vi "new-id.vi"(8 "error in (no error)":errorcluster, 10 "id-string (\"\": generate new id)":string) -> (0 "error out":errorcluster, 3 "ID out":refnum<class "ID.lvclass">)   [LabVIEW 2020, in "graph.lvlib" / "ID.lvclass"]
uses:
  ID.lvclass
  ID.lvclass/ID.ctl
  support/UUID/UUID.lvclass
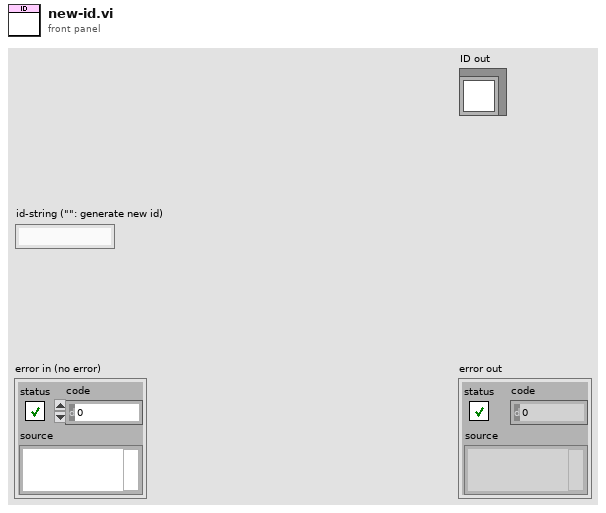
[diagram p1: front panel]
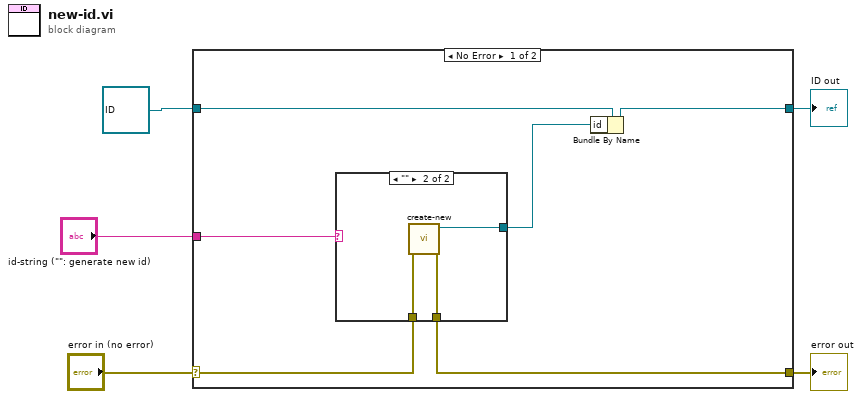
[diagram p0: block diagram]
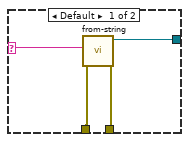
[diagram p2: hidden frame]
diagram:
  n1 = case shown="No Error" "error in (no error)" {
    selector: "error in (no error)" -> [w7 w20]
    tunnel: [w8 w20] -> w4
    tunnel: [w10 w19] -> w2
    tunnel: refnum<class "ID.lvclass"> refnum ("type") -> [w11 w19]
    tunnel: "id-string (\"\": generate new id)" -> [w6 _]
    frame No Error {
      n2 = case shown="\"\"" w6 {
        selector: w6 -> [w13 _]
        tunnel: [w12 w18] -> w9
        tunnel: [w15 w17] -> w8
        tunnel: w7 -> [w14 w16]
        frame Default {
          n3 = call "from-string.vi"("error in (no error)"=w14, "uuid-string"=w13) -> ("error out"=w15:errorcluster, "UUID out"=w12:refnum<class "UUID.lvclass">)  [unwired: 8 in]
        }
        frame "" {
          n4 = call "create-new.vi"("error in (no error)"=w16) -> ("error out"=w17:errorcluster, "UUID out"=w18:refnum<class "UUID.lvclass">)  [unwired: 9 in]
        }
      }
      n5 = Bundle By Name(cluster=w11, "id"=w9) -> (w10:refnum<class "ID.lvclass">)
    }
    frame Error {
    }
  }
  "error out" <- w4
  "ID out" <- w2
